vi "SaveExpParams.vi"(9 "Params":variant, 10 "Full Scan Name":string, 11 "Raw Data Folder":path) -> ()   [LabVIEW 2015]
uses:
  Controls/Spinal Column/spinal_column.ctl
  6733_Red_MOT/6733_control_panel.ctl
  6733_Red_MOT/6733_waveform_parameter_array.ctl
  6733_Red_MOT/6733_waveform_item.ctl
  6733_Red_MOT/Neutral_voltage_conversion_control.ctl
  Controls/6713/6713_waveform_generation.ctl
  Controls/6713/6713_waveform_parameter_array.ctl
  Controls/6713/6713_static_waveform_item.ctl
  Controls/PulseBlaster/Instructions_Cluster.ctl
  Neutral_DAQ/6221 arb waveforms/6221_panel.ctl
  Neutral_DAQ/6221 arb waveforms/6221_waveform_param.ctl
  Controls/Agilent E3631A/Settings_Control.ctl
  Controls/PixelFly/Camera_Initialization.ctl
  Controls/ScanParameters/ScanParametersPanel.ctl
  Controls/ScanParameters/ParameterToChange.ctl
  Controls/ScanParameters/ROI_set.ctl
  Controls/ScanParameters/ScanPBandParam.ctl
  Controls/PicoScope/pico_control_panel.ctl
  Controls/PicoScope/pico_channel_settings.ctl
  Controls/PicoScope/pico_trigger.ctl
  Controls/PicoScope/pico_init_settings.ctl
  Controls/PulseBlaster/delay_control_3..ctl
  Controls/6229/6229_arb_waveform_generation.ctl
  Controls/Synth_409b/Synth_controls.ctl
  Controls/Synth_409b/synth_channel.ctl
  Controls/Synth_409b/table_mode.ctl
  <vilib>/Utility/xml.llb/Write to XML File(string).vi
panel:
  in  "Spinal Column In":T1 {"Red MOT 88 Inputs"."Phase Times" format="%.0p"; "Red MOT 88 Inputs"."Waveform Parameters"."Degree" min=1; "6713 Blue MOT"."Phase Times" format="%.3f"; "Instructions"."Time (s)" min=5e-08 format="%.2p"; "Instructions"."Op Code" items=["Continue", "Stop", "Loop", "End Loop", "JSR", "RTS", "Go To", "Long Delay", "Wait"]; "Instructions"."Instruct Data" format="%#.2p"; "Red MOT 87 Inputs"."Phase Times" format="%.0p"; "Red MOT 87 Inputs"."Waveform Parameters"."Degree" min=1; "ODT Params"."Evaporation Channel" min=0.0 max=1.0 step=1.0; "ODT Params"."Evaporation Phase" min=0.0 max=4.0 step=1.0; "ODT Params"."Phase Times (s)" format="%#_6p"; "Agilent E3631A Settings"."Current Set (1A max)" format="%.3g"; "Agilent E3631A Settings"."Voltage Set (25V max)" format="%.3g"; "Agilent E3631A Settings"."Current Set (5A max)" format="%.3g"; "Agilent E3631A Settings"."Voltage Set (6V max)" format="%.3g"; "PixelFly Initialization"."Bit depth" items=["2"=1]; "PixelFly Initialization"."H bin" items=["1", "2"]; "PixelFly Initialization"."V bin" items=["1", "2"]; "PixelFly Initialization"."boardid in" min=0 max=3 step=1; "PixelFly Initialization"."gain" items=["Low (X1)", "High (X2)"]; "PixelFly Initialization"."exp level" min=0 max=255 step=1; "PixelFly Initialization"."exp time" min=1 max=10000; "PixelFly Initialization"."Exposure mode" items=["Asynch shutter", "Double shot", "Video mode", "Auto exposure"]; "Scan Parameters"."Drop Time (ms)" min=1.0; "Scan Parameters"."Number of Parameters to Scan" min=1; "PicoScope"."Acquisition Settings"."Resolution (s)" min=8e-09 max=34.36 step=8e-09 format="%#_6p"; "PicoScope"."Acquisition Settings"."Post Trigger Time (s)" min=0.0 format="%#_6p"; "PicoScope"."Acquisition Settings"."Pre Trigger Time (s)" min=0.0 format="%#_6p"; "PicoScope"."Pico Scope Inititalization Settings"."Resolution" items=["8-bit", "12-bit", "14-bit", "15-bit (max. 2 ch.)", "16-bit (max. 1 ch.)"]; "PicoScope"."Trigger Options"."Trigger Slope" items=["Rising"=2, "Falling"=3]; "PicoScope"."Channel B Settings"."Range" items=["10 mV", "20 mV", "50 mV", "100 mV", "200 mV", "500 mV", "1 V", "2 V", "5 V", "10 V", "20 V", "50 V ", "100 V"]; "PicoScope"."Channel B Settings"."Coupling" items=["AC", "DC"]; "PicoScope"."Channel A Settings"."Range" items=["10 mV", "20 mV", "50 mV", "100 mV", "200 mV", "500 mV", "1 V", "2 V", "5 V", "10 V", "20 V", "50 V ", "100 V"]; "PicoScope"."Channel A Settings"."Coupling" items=["AC", "DC"]; "Ramp Delay Settings"."Subroutine A"."Time (s)" min=5e-08 format="%.2p"; "Ramp Delay Settings"."Subroutine A"."Op Code" items=["Continue", "Stop", "Loop", "End Loop", "JSR", "RTS", "Go To", "Long Delay", "Wait"]; "Ramp Delay Settings"."Subroutine A"."Instruct Data" format="%#.2p"; "Ramp Delay Settings"."Insert after instruction" min=0; "Ramp Delay Settings"."Delay Step (s)" min=5e-08 format="%#_6p"; "Ramp Delay Settings"."Final Delay Time (s)" min=5e-08 format="%#_6p"; "Ramp Delay Settings"."Initial Delay Time (s)" min=5e-08 format="%#_6p"; "6229 Green Lattice Inputs"."Phase Times" format="%.3f"; "6229 Green Lattice Inputs"."Waveform Parameters"."Degree" min=1}
  # "Channel 0"
  # "Channel 1"
  # "Channel 2"
  # "Channel 3"
  # "Channel 4"
  # "Channel 5"
  # "Channel 7"
  # "Channel 7"
  # "(0) 689 Center Freq"
  # "(1) 689 Dither Amp"
  # "(2) 689 Power Lock"
  # "(3) Red MOT Field Grad"
  # "Channel 0"
  # "Channel 1"
  # "Channel 2"
  # "Channel 3"
  # "Channel 4"
  # "Channel 5"
  # "Channel 7"
  # "Channel 7"
  # "6V Output Settings"
  # "25V Output Settings"
  # "Select a PB Channel to set with a phase time\nfor evaporation or whatever"
  # "(0) Arm A"
  # "(1) Arm B"
  # "(2) Arm C"
  # "(3) Unused"
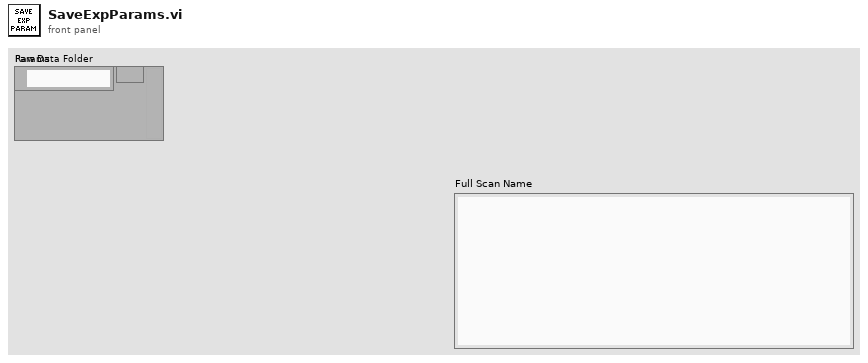
[diagram p1: front panel]
types:
  T1 = typedef "spinal_column.ctl" = cluster{"Red MOT 88 Inputs":T2, "6713 Blue MOT":T6, "Instructions":T9, "Red MOT 87 Inputs":T2, "ODT Params":T10, "Agilent E3631A Settings":T12, "PixelFly Initialization":T13, "Scan Parameters":T14, "PicoScope":T18, "Ramp Delay Settings":T22, "6229 Green Lattice Inputs":T23, "Synth Controls 1":T24, "Synth Controls 2":T24, "Control Reference Cluster":cluster{"Controls[]":refnum<vi>[], "Control Names":string[]}}
  T2 = typedef "6733_control_panel.ctl" = cluster{"Active Device":string, "Active Channels":bool[], "Waveform Parameters":T3, "Active Phases":bool[], "Phase Times":dbl[], "Trigger Channel":tag}
  T3 = typedef "6733_waveform_parameter_array.ctl" = T4[][]
  T4 = typedef "6733_waveform_item.ctl" = cluster{"Function":enum16{"Polynomial", "Exponential", "Constant"}, "Initial":dbl, "Final":dbl, "Degree":i8, "Nickname":string, "Conversion":T5, "Constant":dbl}
  T5 = typedef "Neutral_voltage_conversion_control.ctl" = enum16{"Volts", "B Field Grad (G/cm)", "Red MOT Center Freq (MHz)", "Red Dither Pk(kHz)", "Red Power (mW)", "ODT Sheet Trap Power (W)", "ODT Loading Trap Power (W)"}
  T6 = typedef "6713_waveform_generation.ctl" = cluster{"Active Device":string, "Active Channels":bool[], "Waveform Parameters":T7, "Active Phases":bool[], "Phase Times":dbl[], "Trigger Channel":tag, "FIFO Buffer Size":dbl}
  T7 = typedef "6713_waveform_parameter_array.ctl" = T8[][]
  T8 = typedef "6713_static_waveform_item.ctl" = cluster{"Constant":dbl, "Nickname":string, "Conversion":T5}
  T9 = typedef "Instructions_Cluster.ctl" = cluster{"Instruct Data":i32, "Op Code":i32, "Flags":bool[], "Comments":string, "Time (s)":dbl, "Column Number":string, "Array":string[]}[]
  T10 = typedef "6221_panel.ctl" = cluster{"Waveform Parameters":T11[][], "Active Phases":bool[], "Active Channels":bool[], "Phase Times (s)":dbl[], "Active Device":string, "Trigger Channel":tag, "Evaporation Phase":dbl, "Evaporation Channel":dbl}
  T11 = typedef "6221_waveform_param.ctl" = cluster{"Initial Value":dbl, "Final Value":dbl, "Tau":dbl, "Eta":dbl, "Nickname":string, "Enum":enum16{"Power Law", "Evaporation Formula"}, "Conversion":T5}
  T12 = typedef "Settings_Control.ctl" = cluster{"VISA resource name":refnum<visa-resource-name>, "Voltage Set (6V max)":dbl, "Current Set (5A max)":dbl, "Voltage Set (25V max)":dbl, "Current Set (1A max)":dbl}
  T13 = typedef "Camera_Initialization.ctl" = cluster{"Exposure mode":u16, "exp time":i32, "exp level":i32, "gain":i32, "boardid in":i32, "offset":i32, "V bin":i32, "H bin":i32, "trigger":bool, "Bit depth":i32}
  T14 = typedef "ScanParametersPanel.ctl" = cluster{"Initial Values":dbl[], "Final Values":dbl[], "Step Sizes":dbl[], "Parameters to Change":T15[], "Channels to Change":dbl[], "Number of Parameters to Scan":i32, "Parameter Nickname (no spaces)":string[], "Scan Base Name":string, "Raw_Data Folder":path, "ROI Parameters":T16, "Drop Time (ms)":dbl, "ODT VCA 1 Channel":dbl, "ODT VCA 2 Channel":dbl, "Phases To Change":dbl[], "Scan Pulseblaster Channel With Parameter":T17, "Preserve Waveform\nContinuity":bool, "Generated Array Type":enum16{"Custom Array From File", "Default (old way)"}, "Principle Quantum #":i32, "Angular Momentum":enum16{"s", "p", "d", "f", "g", "h"}, "Ramp Delay Channel":i32, "ODT Hold Channel":i32, "MCS ROI Min":i32, "MCS ROI Max":i32, "Master Batch Fourth Column":dbl}
  T15 = typedef "ParameterToChange.ctl" = enum16{"Delay single delay time", "Dummy Variable", "Delay Exposure", "PB Loops", "Number of Delay Loops", "Subroutine A Time", "Subroutine B Time", "Synth Amplitude", "Synth Frequency", "Synth Phase", "ODT Params Phase Time", "ODT Params Tau", "ODT Params Final Voltage", "ODT Params Initial Voltage", "ODT Params Eta", "Red Mot 88 Phase Time", "Red Mot 87 Phase Time", "Red Mot 88 Final Voltage", "Red Mot 88 Initial Voltage", "Red Mot 87 Final Voltage", "Red Mot 87 Initial Voltage", "PulseBlaster", "6713 Voltage"}
  T16 = typedef "ROI_set.ctl" = cluster{"Background Radius":dbl, "Atom Radius":dbl, "X Center":dbl, "Y Center":dbl}
  T17 = typedef "ScanPBandParam.ctl" = cluster{"Change PB Time Toggle":bool, "PB Channel":dbl, "Parameter Number":dbl}
  T18 = typedef "pico_control_panel.ctl" = cluster{"Channel A Settings":T19, "Channel B Settings":T19, "Trigger Options":T20, "Pico Scope Inititalization Settings":T21, "Use PicoScope?":bool, "Acquisition Settings":cluster{"Pre Trigger Time (s)":dbl, "Post Trigger Time (s)":dbl, "Resolution (s)":dbl, "Four Channel Device":bool, "Number of Captures":dbl}}
  T19 = typedef "pico_channel_settings.ctl" = cluster{"Enabled":bool, "Coupling":i16, "Range":u16, "Analogue Offset":sgl}
  T20 = typedef "pico_trigger.ctl" = cluster{"Trigger Enabled":bool, "Trigger Source":enum16{"Channel A", "Channel B", "Channel C", "Channel D", "Ext."}, "Trigger Threshold (-5 to 5 V)":dbl, "Trigger Slope":u16, "Trigger Delay (ms)":dbl, "Auto Trigger Time (ms)":i16}
  T21 = typedef "pico_init_settings.ctl" = cluster{"USB Power":bool, "Use Serial Number":bool, "Resolution":i32, "Serial Number":string, "Handle":i16}
  T22 = typedef "delay_control_3..ctl" = cluster{"Insert Delays":bool, "Number of loops":i32, "Insert after instruction":i32, "Random":bool, "Initial Delay Time (s)":dbl, "Final Delay Time (s)":dbl, "Delay Step (s)":dbl, "Delay Column":dbl, "Loop Hold Column":dbl, "Field Ramp Column":dbl, "Excitation Column":dbl, "Hold + Delay + Excitation Time":dbl, "Ascending/Descending":bool, "Subroutine A":T9}
  T23 = typedef "6229_arb_waveform_generation.ctl" = cluster{"Active Device":string, "Active Channels":bool[], "Waveform Parameters":T3, "Active Phases":bool[], "Phase Times":dbl[], "Trigger Channel":tag, "FIFO Buffer Size":dbl}
  T24 = typedef "Synth_controls.ctl" = cluster{"Channel Settings":T25[], "Active Channels":bool[], "COM Port":refnum<visa-resource-name>, "Table Mode":T26}
  T25 = typedef "synth_channel.ctl" = cluster{"Voltage (Amp.) ":dbl, "Frequency (MHz)":dbl, "Phase (deg)":dbl, "Nickname":string}
  T26 = typedef "table_mode.ctl" = cluster{"Table Mode On/Off":bool, "Initial Frequency (MHz)":dbl, "FinalFreq":dbl, "Frequency Step (MHz)":dbl, "Ascending/Descending":bool, "Random":bool}
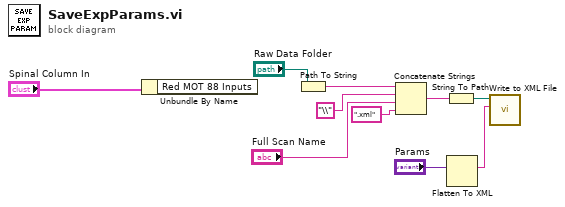
[diagram p0: block diagram]
diagram:
  n1 = Unbundle By Name("Spinal Column In") -> ()  [unwired: 1 out]
  n2 = Path To String(path="Raw Data Folder") -> (string=w4:string)
  n3 = Concatenate Strings(w4, "\\" ("string"), "Full Scan Name", ".xml") -> (w8:string)
  n4 = String To Path(string=w8) -> (path=w7:path)
  n5 = Flatten To XML(anything="Params") -> (xml string=w6:string)
  n6 = call-poly <vilib>:"Write to XML File.vi"("XML Input"=w6, "XML File Path"=w7) -> ()  [unwired: 7 in, 3 out]
